vi "Image Merge Axes.vi"(0 "Image In":dbl[][](array[numeric]), 5 "CCD Area Format":T1) -> (4 "Image Out":dbl[][](array[numeric]))   [LabVIEW 2010]
uses:
  Symphony/TypeDefs/Symphony Area Format.ctl
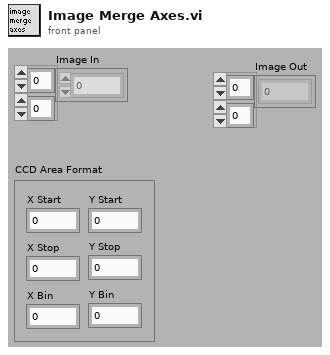
[diagram p1: front panel]
types:
  T1 = typedef "Symphony Area Format.ctl" = cluster{"XStart":i32, "YStart":i32, "XStop":i32, "YStop":i32, "XBin":i32, "YBin":i32}
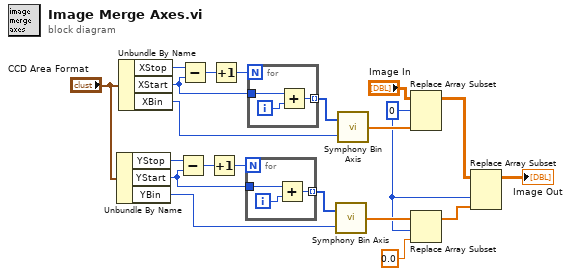
[diagram p0: block diagram]
diagram:
  w1 = 0 ("index (row)")
  n1 = Unbundle By Name("CCD Area Format") -> ("YStop"=w12:i32, "YStart"=w11:i32, "YBin"=w5:i32)
  n2 = Unbundle By Name("CCD Area Format") -> ("XStop"=w16:i32, "XStart"=w15:i32, "XBin"=w8:i32)
  n3 = Subtract(x=w12, y=w11) -> (x-y=w14:i32)
  n4 = Subtract(x=w16, y=w15) -> (x-y=w18:i32)
  n5 = Increment(x=w14) -> (x+1=w13:i32)
  n6 = Increment(x=w18) -> (x+1=w17:i32)
  n7 = for {
    N: w13 -> [_]
    tunnel: w11 -> [w23]
    tunnel: [w22] -> w6 mode=indexing
    i -> [w24]
    n8 = Add(x=w23, y=w24) -> (x+y=w22:i32)
  }
  n9 = for {
    N: w17 -> [_]
    tunnel: w15 -> [w26]
    tunnel: [w25] -> w9 mode=indexing
    i -> [w27]
    n10 = Add(x=w26, y=w27) -> (x+y=w25:i32)
  }
  n11 = call "Symphony Bin Axis.vi"("Binning Factor"=w5, "Axis In"=w6) -> ("Axis Out"=w4:dbl[])
  n12 = call "Symphony Bin Axis.vi"("Binning Factor"=w8, "Axis In"=w9) -> ("Axis Out"=w7:dbl[])
  n13 = Replace Array Subset(array="Image In", new element=w7, index (row)=w1) -> (w20:dbl[][])  [unwired: 1 in]
  n14 = Replace Array Subset(array=w4, new element=0.0 ("new element/subarray"), index=w1) -> (w2:dbl[])
  n15 = Replace Array Subset(array=w20, new element=w2, index (col)=w1) -> (→"Image Out":dbl[][])  [unwired: 1 in]
